vi "MSDateienSchicken12-15.vi"(1 "MSNummer":i32, 2 "MSa?":bool=TRUE, 3 "Dateipfad:fromcriordy":path, 4 "Dateipfad:fromcriocmd":path) -> ()   [LabVIEW 2017]
uses:
  GVZeitenZyklen.vi
  GVProbenvol.vi
  GVVentilposition.vi
  <vilib>/FTP/NI_FTP.lvlib
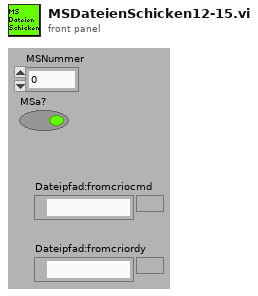
[diagram p1: front panel]
types:
  T1 = enum16{"open", "replace", "create", "open or create", "replace or create", "replace or create with confirmation"}
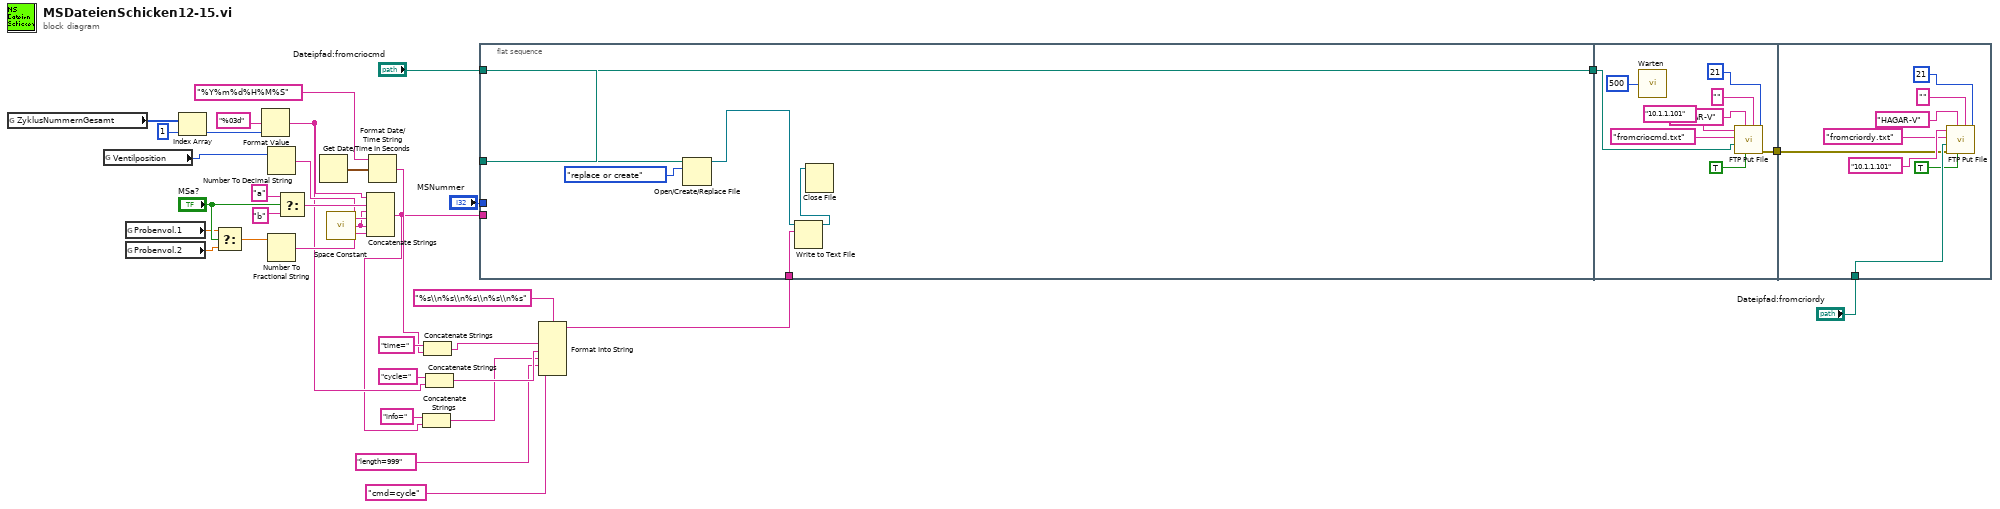
[diagram p0: block diagram]
diagram:
  n1 = global read "GVZeitenZyklen.vi" "ZyklusNummernGesamt"() -> (w30:i32[])
  n2 = global read "GVVentilposition.vi" "Ventilposition"() -> (w14:i32)
  n3 = global read "GVProbenvol.vi" "Probenvol.1"() -> (w16:dbl)
  n4 = global read "GVProbenvol.vi" "Probenvol.2"() -> (w15:dbl)
  n5 = Index Array(array=w30, index=1 ("Index")) -> (element=w26:i32)
  n6 = Select(t=w16, s="MSa?", f=w15) -> (s? t:f=w18:dbl)
  n7 = Format Value(format string="%03d" ("Format-String"), value (0)=w26) -> (output string=w8:string)  [unwired: 1 in]
  n8 = Number To Decimal String(number=w14) -> (decimal integer string=w21:string)  [unwired: 1 in]
  n9 = Number To Fractional String(number=w18) -> (F-format string=w17:string)  [unwired: 3 in]
  n10 = Select(t="a", s="MSa?", f="b") -> (s? t:f=w22:string)
  n11 = Get Date/Time In Seconds() -> (seconds since 1Jan1904=w32:timestamp)
  n12 = call <vilib>:"Space Constant.vi"() -> ("String"=w20:string)
  n13 = Concatenate Strings(w8, w22, w20, w21, w20, w17) -> (w5:string)
  n14 = Format Date/Time String(time format string (%c)="%Y%m%d%H%M%S" ("Zeitformatierungs-String (%c)"), seconds (now)=w32) -> (date/time string=w11:string)  [unwired: 1 in]
  n15 = Concatenate Strings("info=" ("string"), w5) -> (w4:string)
  n16 = Concatenate Strings("time=" ("string"), w11) -> (w10:string)
  n17 = Concatenate Strings("cycle=" ("string"), w8) -> (w7:string)
  n18 = flat-sequence {
    tunnel: [w41] -> w28
    tunnel: w5 -> [_]
    tunnel: "MSNummer" -> [_]
    tunnel: "Dateipfad:fromcriocmd" -> [w41]
    tunnel: "Dateipfad:fromcriocmd" -> [w40]
    tunnel: w1 -> [w36]
    tunnel: [w42] -> w27
    tunnel: w28 -> [w47]
    tunnel: "Dateipfad:fromcriordy" -> [w55]
    tunnel: w27 -> [w51]
    frame #0 {
      n19 = Open/Create/Replace File(file path (use dialog)=w40, operation (0:open)=T1."replace or create" ("Operation (0:Öffnen)")) -> (refnum out=w38:refnum<file>)  [unwired: 4 in, 2 out]
      n20 = Write to Text File(file (use dialog)=w38, text=w36) -> (refnum out=w37:refnum<file>)  [unwired: 2 in, 2 out]
      n21 = Close File(refnum=w37) -> ()  [unwired: 1 in, 2 out]
    }
    frame #1 {
      n22 = call "Warten"("Count(mSec)"=u32 500 ("Zu wartende ms")) -> ()  [unwired: 1 out]
      n23 = call <vilib>:"FTP Put File.vi"("remote port (21)"=u16 21, "password"="" ("user"), "binary (F)"=TRUE, "user"="HAGAR-V", "local path"=w47, "remote path"="fromcriocmd.txt", "host"="10.1.1.101") -> ("error out"=w42:errorcluster)  [unwired: 3 in, 1 out]
    }
    frame #2 {
      n24 = call <vilib>:"FTP Put File.vi"("remote port (21)"=u16 21, "password"="" ("user"), "binary (F)"=TRUE, "user"="HAGAR-V", "error in (no error)"=w51, "local path"=w55, "remote path"="fromcriordy.txt", "host"="10.1.1.101") -> ()  [unwired: 2 in, 2 out]
    }
  }
  n25 = Format Into String(format string="%s\\n%s\\n%s\\n%s\\n%s", w10, w7, w4, "length=999" ("string"), "cmd=cycle" ("string")) -> (resulting string=w1:string)  [unwired: 2 in, 1 out]
